vi "Animate.vi"(4 "heading":dbl, 5 "xy_position":dbl[](array[numeric])=[0.0, 0.0], 6 "error in (no error)":errorcluster, 7 "Steer Angle":dbl, 8 "Car Speed":dbl, 9 "task in":refnum<class "Visualization.lvclass">) -> (0 "slope":dbl, 2 "error out":errorcluster, 3 "task out":refnum<class "Visualization.lvclass">)   [LabVIEW 2018]
uses:
  <vilib>/Quanser/Rapid Control Prototyping Toolkit/visualization/Visualization.lvclass
  <vilib>/Quanser/Rapid Control Prototyping Toolkit/sources/CL Sample Time.vi
  <vilib>/Simulation/Implementation/Shared/SIMSCR Execution Mode.ctl
  <vilib>/Simulation/Scripting/Companion Diagram/SimConfigNode/SimParams.ctl
  <vilib>/Simulation/Scripting/Companion Diagram/SimConfigNode/_simSolvers.ctl
  <vilib>/Simulation/Param Hierarchy/Typedefs/SIMPH Param Control Actions.ctl
  <vilib>/Simulation/Implementation/Shared/NILVSim_ParamChanged.vi
  <vilib>/Simulation/Implementation/Shared/NILVSIM_BeginStep.vi
  <vilib>/Simulation/SignalArithmetic/Implementation/NILVSim Gain.llb/SIM Gain (scalar).vi
  <vilib>/Simulation/Utility/Implementation/NILVSim Memory.llb/NILVSim Memory (core).vi
  <vilib>/Simulation/Implementation/Shared/NILVSim_Manager.vi
  <vilib>/Utility/error.llb/Clear Errors.vi
  <vilib>/Simulation/Implementation/Shared/NILVSim_FinalizeModel.vi
  <vilib>/Simulation/Implementation/Shared/SIM Unbundle Sim Info.vi
  <vilib>/Simulation/Implementation/Shared/SIMSH Read Queue.vi
  <vilib>/Simulation/Implementation/Shared/NILVSim_Initialize.vi
  <vilib>/imath/engines/lvmath2/RunTimeEngine/IndexRead/NIMS V(S).vi
  <instcachedir>/0/NIMS V(S)_0488751826AF41519A22953C041130DC.lvgen/NIMS V(S)_0488751826AF41519A22953C041130DC_000.vi
  <vilib>/imath/engines/lvmath2/RunTimeEngine/ErrorHandling/NIMS_Create Error From Enums.vi
  <vilib>/imath/engines/lvmath2/RunTimeEngine/ArithmeticOperatorToken/NIMS_ArithmeticOperator_multmx(M,CV)-internal.vi
  <instcachedir>/0/NIMS_ArithmeticOperator_multmx(M,CV)-internal_5287250D8D1D4A3E9F77F5DF08D432E0.lvgen/NIMS_ArithmeticOperator_multmx(M,CV)-internal_5287250D8D1D4A3E9F77F5DF08D432E0_002.vi
  <vilib>/imathl/engines/lvmath/Functions/Error Handling/Create Error.vi
  <vilib>/imath/engines/lvmath2/RunTimeEngine/BuiltInFunctions/atan2/NIMS_atan2.vi
  <instcachedir>/0/NIMS_atan2_A91AA4A7D42247EDBE8F76DB99AF04A4.lvgen/NIMS_atan2_A91AA4A7D42247EDBE8F76DB99AF04A4_000.vi
  <vilib>/imath/engines/lvmath2/RunTimeEngine/ArithmeticOperatorToken/NIMS_ArithmeticOperator_multmx-internal.vi
  <instcachedir>/0/NIMS_ArithmeticOperator_multmx-internal_16A6E1DA326644AB974D30232E729C42.lvgen/NIMS_ArithmeticOperator_multmx-internal_16A6E1DA326644AB974D30232E729C42_004.vi
  <instcachedir>/0/NIMS_ArithmeticOperator_multmx-internal_16A6E1DA326644AB974D30232E729C42.lvgen/NIMS_ArithmeticOperator_multmx-internal_16A6E1DA326644AB974D30232E729C42_000.vi
  <vilib>/imath/engines/lvmath2/RunTimeEngine/IndexRead/NIMS V(R2).vi
  <instcachedir>/0/NIMS V(R2)_C76619605A0E4E9F8B2FA9389712AC47.lvgen/NIMS V(R2)_C76619605A0E4E9F8B2FA9389712AC47_002.vi
  <vilib>/imath/engines/lvmath2/RunTimeEngine/IndexReplace/NIMS M(R2,S)=V.vi
  <instcachedir>/0/NIMS M(R2,S)=V_54A43CB67E254D00A7B7B97DBD1A234B.lvgen/NIMS M(R2,S)=V_54A43CB67E254D00A7B7B97DBD1A234B_000.vi
  <vilib>/imath/engines/lvmath2/RunTimeEngine/IndexRead/NIMS M(R2,S).vi
  <instcachedir>/0/NIMS M(R2,S)_56813DCFDD5A484292D2195AF15D2BF5.lvgen/NIMS M(R2,S)_56813DCFDD5A484292D2195AF15D2BF5_000.vi
  <vilib>/imath/engines/lvmath2/RunTimeEngine/NodeEndStatement/NIMS_NodeEndStatement_Output.vi
  <instcachedir>/0/NIMS_NodeEndStatement_Output_53EC0D466D134D7ABD903AC30B43404B.lvgen/NIMS_NodeEndStatement_Output_53EC0D466D134D7ABD903AC30B43404B_001.vi
  <instcachedir>/0/NIMS_NodeEndStatement_Output_53EC0D466D134D7ABD903AC30B43404B.lvgen/NIMS_NodeEndStatement_Output_53EC0D466D134D7ABD903AC30B43404B_002.vi
  <vilib>/imath/engines/lvmath2/RunTimeEngine/ErrorHandling/NIMS_Finalize Error.vi
  <vilib>/Simulation/Utility/Implementation/NILVSim Get Time and IsAcceptedStep.vi
  <instcachedir>/0/NIMS_NodeEndStatement_Output_53EC0D466D134D7ABD903AC30B43404B.lvgen/NIMS_NodeEndStatement_Output_53EC0D466D134D7ABD903AC30B43404B_005.vi
  <vilib>/Quanser/Rapid Control Prototyping Toolkit/visualization/Visualization Set Variable (1D SGL).vi
  <vilib>/Quanser/Rapid Control Prototyping Toolkit/visualization/Visualization Set Variable (2D SGL).vi
  <vilib>/Simulation/Implementation/Shared/NILVSim_GetModelError.vi
  <vilib>/Simulation/Implementation/Shared/SIM SimErrorHandler.vi
  <vilib>/Simulation/Implementation/Shared/SIM Bundle Sim Info.vi
  <vilib>/Simulation/Scripting/Companion Diagram/SimConfigNode/SimDog.xnode
  <vilib>/Simulation/Implementation/XNodeFramework/SimXNode/SimX.xnode
  <vilib>/Simulation/Implementation/Shared/NI_SIM_Implementation.lvlib
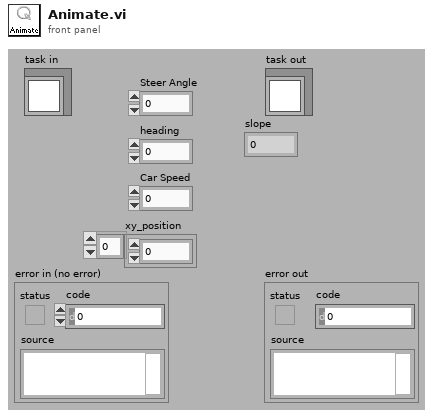
[diagram p1: front panel]
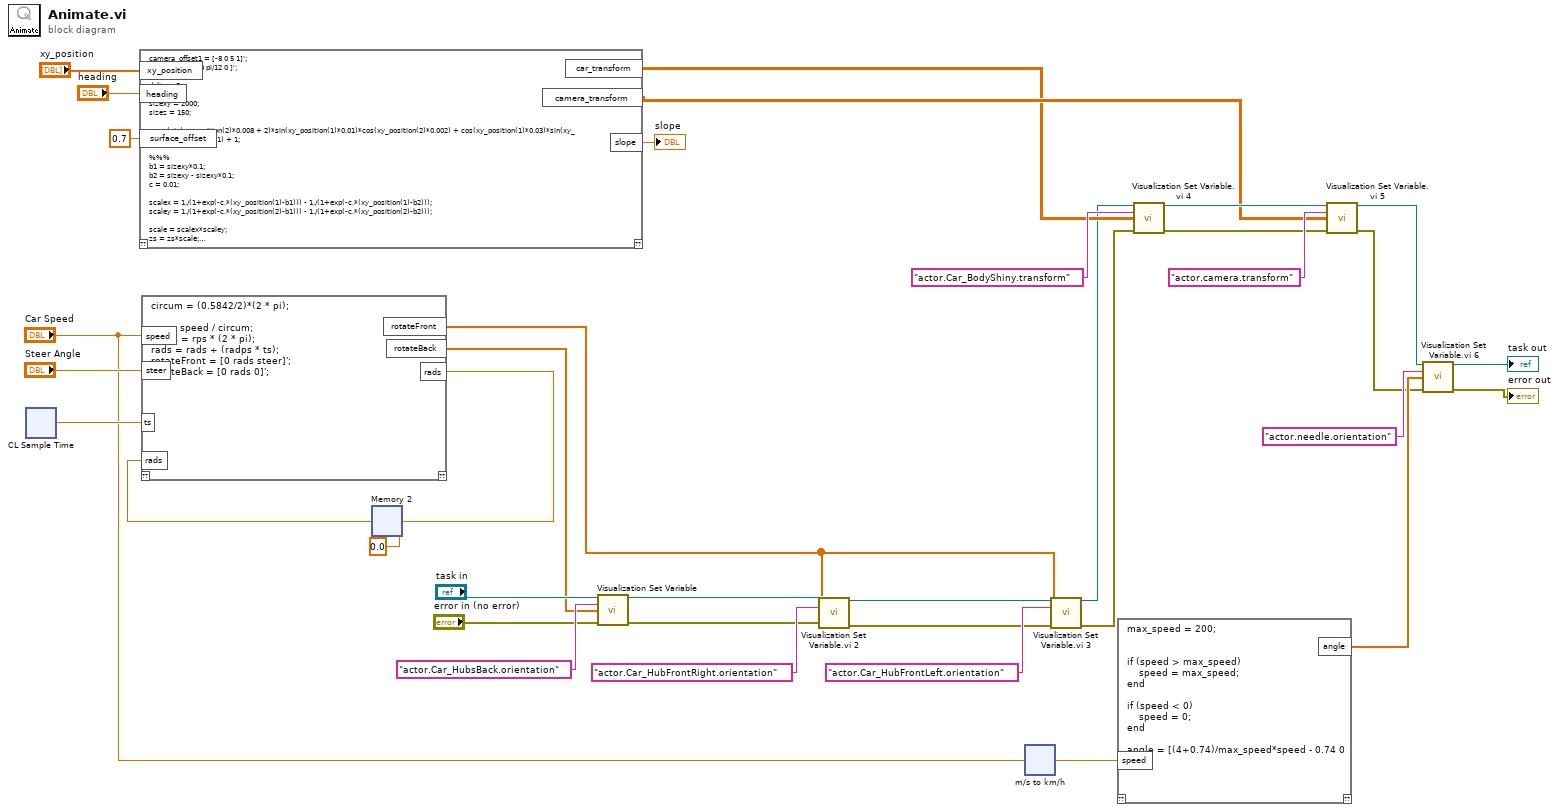
[diagram p0: block diagram]
diagram:
  n1 = xnode "CL Sample Time"() -> ("time (seconds)"=w17:dbl)
  n2 = mathscript code="camera_offset1 = [-8 0 5 1]';\nviewangle1 = [0 pi/12 0 ]';\n\ndelta = 5;\n\nsizexy = 2000;\nsizez = 150;\n\nzs = (sin(xy_position(2)*0.008 + 2)*sin(xy_position(1)*0.01)*cos(xy_position(2)*0.002) + cos(xy_position(1)*0.03)*sin(xy_position(2)*0.04)*0.1) + 1;\n\n%%%\nb1 = sizexy*0.1;\nb2 = sizexy - sizexy*0.1;\nc = 0.01;\n\nscalex = 1./(1+exp(-c.*(xy_position(1)-b1))) - 1./(1+exp(-c.*(xy_position(1)-b2)));\nscaley = 1./(1+exp(-c.*(xy_position(2)-b1))) - 1./(1+exp(-c.*(xy_position(2)-b2)));\n\nscale = scalex*scaley;\nzs = zs*scale;\n\nzs = zs*0.5*sizez;\n\nvecN = [delta 0]';\nvecE = [0 delta]';\n\nrot_z = [cos(heading) -sin(heading); sin(heading) cos(heading)];\nvecN = rot_z*vecN;\nvecE = rot_z*vecE;\n\n%%%%\nzN = (sin((vecN(2) + xy_position(2))*0.008 + 2)*sin((vecN(1) + xy_position(1))*0.01)*cos((vecN(2) + xy_position(2))*0.002) + cos((vecN(1) + xy_position(1))*0.03)*sin((vecN(2) + xy_position(2))*0.04)*0.1) + 1;\n\nscalex = 1./(1+exp(-c.*((vecN(1) + xy_position(1))-b1))) - 1./(1+exp(-c.*((vecN(1) + xy_position(1))-b2)));\nscaley = 1./(1+exp(-c.*((vecN(2) + xy_position(2))-b1))) - 1./(1+exp(-c.*((vecN(2) + xy_position(2))-b2)));\n\nscale = scalex*scaley;\nzN = zN*scale;\nzN = zN*0.5*sizez;\n\n%%%%\nzE = (sin((vecE(2) + xy_position(2))*0.008 + 2)*sin((vecE(1) + xy_position(1))*0.01)*cos((vecE(2) + xy_position(2))*0.002) + cos((vecE(1) + xy_position(1))*0.03)*sin((vecE(2) + xy_position(2))*0.04)*0.1) + 1;\n\nscalex = 1./(1+exp(-c.*((vecE(1) + xy_position(1))-b1))) - 1./(1+exp(-c.*((vecE(1) + xy_position(1))-b2)));\nscaley = 1./(1+exp(-c.*((vecE(2) + xy_position(2))-b1))) - 1./(1+exp(-c.*((vecE(2) + xy_position(2))-b2)));\n\nscale = scalex*scaley;\nzE = zE*scale;\nzE = zE*0.5*sizez;\n%%%%\n\nrx = atan2(zE-zs, delta);\nry = -atan2(zN-zs, delta);\n%%%%%\n\nz = zs;\n\nrot_x = [1 0 0 0; 0 cos(rx) -sin(rx) 0; 0 sin(rx) cos(rx) 0; 0 0 0 1];\nrot_y = [cos(ry) 0 sin(ry) 0; 0 1 0 0; -sin(ry) 0 cos(ry) 0; 0 0 0 1];\nrot_z = [cos(heading) -sin(heading) 0 0; sin(heading) cos(heading) 0 0; 0 0 1 0; 0 0 0 1];\n\noverhead_view = ([1 0 0 xy_position(1); 0 1 0 xy_position(2); 0 0 1 z+5; 0 0 0 1]*rot_z*rot_y*rot_x)*[20 0 0 0; 0 20 0 0; 0 0 20 0; 0 0 0 1];\ncar_transform = [1 0 0 xy_position(1); 0 1 0 xy_position(2); 0 0 1 z+surface_offset; 0 0 0 1]*rot_z*rot_y*rot_x;\n\nrot_x_view1 = [1 0 0 0; 0 cos(viewangle1(1)) -sin(viewangle1(1)) 0; 0 sin(viewangle1(1)) cos(viewangle1(1)) 0; 0 0 0 1];\nrot_y_view1 = [cos(viewangle1(2)) 0 sin(viewangle1(2)) 0; 0 1 0 0; -sin(viewangle1(2)) 0 cos(viewangle1(2)) 0; 0 0 0 1];\nrot_z_view1 = [cos(viewangle1(3)) -sin(viewangle1(3)) 0 0; sin(viewangle1(3)) cos(viewangle1(3)) 0 0; 0 0 1 0; 0 0 0 1];\nbackview_transform = rot_z_view1*rot_y_view1*rot_x_view1;\nbackview_transform(1:3,4) = camera_offset1(1:3);\ncamera_transform = [1 0 0 xy_position(1); 0 1 0 xy_position(2); 0 0 1 z+surface_offset; 0 0 0 1]*rot_z*backview_transform;\ncam_pos = camera_transform(1:3,4);\n\n%filter_weight = 0.05;\ncam_pos_filtered = cam_pos; %last_pos*(1.0 - filter_weight) + filter_weight*cam_pos;\n%last_pos = cam_pos_filtered;\n\ncamera_transform(1:3,4) = cam_pos_filtered;\ncar_transform = car_transform';\ncamera_transform = camera_transform';\nslope = -ry;" ("MathScript Node 3")("xy_position"="xy_position", "heading"="heading", "surface_offset"=0.7) -> ("car_transform"=w8:dbl[][], "camera_transform"=w9:dbl[][], "slope"=→"slope":dbl)  [unwired: 1 in, 1 out]
  n3 = xnode "m/s to km/h"("input"="Car Speed") -> ("output"=w2:dbl)  [unwired: 3 in]
  n4 = mathscript code="max_speed = 200;\n\n\nif (speed > max_speed)\n    speed = max_speed;\nend\n\nif (speed < 0)\n    speed = 0;\nend\n\nangle = [(4+0.74)/max_speed*speed - 0.74 0 0]';"("speed"=w2) -> ("angle"=w14:dbl[])  [unwired: 1 in, 1 out]
  n5 = mathscript code="circum = (0.5842/2)*(2 * pi);\n\nrps = speed / circum;\nradps = rps * (2 * pi);\nrads = rads + (radps * ts);\nrotateFront = [0 rads steer]';\nrotateBack = [0 rads 0]';" ("MathScript Node 2")("speed"="Car Speed", "steer"="Steer Angle", "ts"=w17, "rads"=w25) -> ("rotateFront"=w16:dbl[], "rotateBack"=w15:dbl[], "rads"=w27:dbl)  [unwired: 1 in, 1 out]
  n6 = xnode ("Memory 2")("input"=w27, "initial value"=0.0) -> ("output"=w25:dbl)  [unwired: 4 in]
  n7 = call-poly <vilib>:"Visualization Set Variable.vi"("visualization in"="task in", "variable name"="actor.Car_HubsBack.orientation" ("variable name 2"), "values"=w15, "error in (no error)"="error in (no error)") -> ("visualization out"=w31:refnum<class "Visualization.lvclass">, "error out"=w33:errorcluster)  [unwired: 10 in]
  n8 = call-poly "Visualization Set Variable.vi 2"("visualization in"=w31, "variable name"="actor.Car_HubFrontRight.orientation" ("variable name 3"), "values"=w16, "error in (no error)"=w33) -> ("visualization out"=w30:refnum<class "Visualization.lvclass">, "error out"=w32:errorcluster)  [unwired: 10 in]
  n9 = call-poly "Visualization Set Variable.vi 3"("visualization in"=w30, "variable name"="actor.Car_HubFrontLeft.orientation" ("variable name 4"), "values"=w16, "error in (no error)"=w32) -> ("visualization out"=w7:refnum<class "Visualization.lvclass">, "error out"=w6:errorcluster)  [unwired: 10 in]
  n10 = call-poly "Visualization Set Variable.vi 4"("visualization in"=w7, "variable name"="actor.Car_BodyShiny.transform" ("variable name 6"), "values"=w8, "error in (no error)"=w6) -> ("visualization out"=w11:refnum<class "Visualization.lvclass">, "error out"=w10:errorcluster)  [unwired: 10 in]
  n11 = call-poly "Visualization Set Variable.vi 5"("visualization in"=w11, "variable name"="actor.camera.transform", "values"=w9, "error in (no error)"=w10) -> ("visualization out"=w5:refnum<class "Visualization.lvclass">, "error out"=w4:errorcluster)  [unwired: 10 in]
  n12 = call-poly "Visualization Set Variable.vi 6"("visualization in"=w5, "variable name"="actor.needle.orientation" ("variable name 5"), "values"=w14, "error in (no error)"=w4) -> ("visualization out"=→"task out":refnum<class "Visualization.lvclass">, "error out"=→"error out":errorcluster)  [unwired: 10 in]
